vi "PongStrategy.vi"(9 "TargetTile":u16(ring)=36, 10 "Hand":u16[](array[ring])) -> (2 "Pong?":bool)   [LabVIEW 2025]
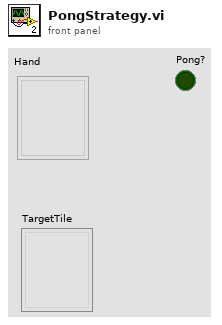
[diagram p1: front panel]
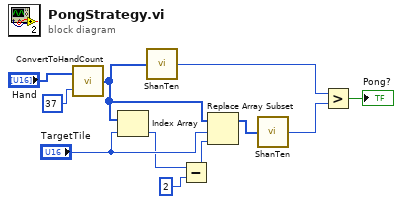
[diagram p0: block diagram]
diagram:
  n1 = call "ConvertToHandCount.vi"("AddtionalTile"=u16 37, "Hand"="Hand") -> ("HandCount"=w8:u16[])
  n2 = Index Array(array=w8, index="TargetTile") -> (element=w5:u16)
  n3 = call "ShanTen.vi"("Count"=w8) -> ("ShanTen"=w3:i16)
  n4 = Subtract(x=w5, y=2) -> (x-y=w6:i32)
  n5 = Replace Array Subset(array=w8, new element=w6, index="TargetTile") -> (w9:u16[])
  n6 = call "ShanTen.vi"("Count"=w9) -> ("ShanTen"=w2:i16)
  n7 = Greater?(x=w3, y=w2) -> (0:→"Pong?":bool)
